vi "ClientTestVI.vi"() -> ()   [LabVIEW 2018, in "TCP_Client.lvlib"]
uses:
  TCP_Client/TCP_Client.lvclass
  TCP_Client.lvlib
panel:
  out "Waveform Graph":dbl[](graph)
  in  "stop":bool
  out "error out":errorcluster
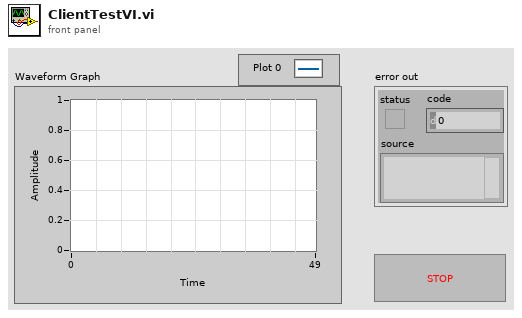
[diagram p1: front panel]
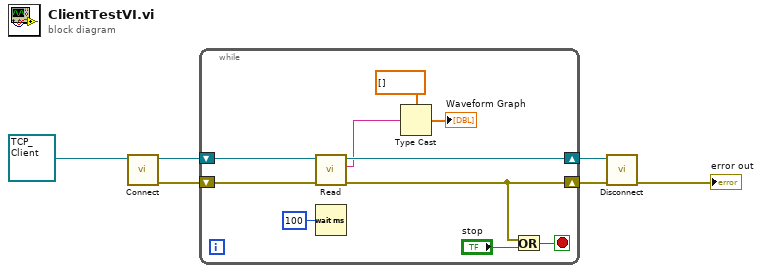
[diagram p0: block diagram]
diagram:
  n1 = call-dynamic "Connect.vi"("TCP_Client in"=refnum<class "TCP_Client.lvclass"> refnum) -> ("error out"=w4:errorcluster, "TCP_Client out"=w5:refnum<class "TCP_Client.lvclass">)  [unwired: 9 in]
  n2 = while {
    shift-right: [w14] -> w3
    shift-left: w5 -> [w16]
    shift-right: [w13] -> w2
    shift-left: w4 -> [w15]
    stop <- w11 stop-if-true
    n3 = call-dynamic "Read.vi"("error in (no error)"=w15, "TCP_Client in"=w16) -> ("error out"=w13:errorcluster, "Message"=w8:string, "TCP_Client out"=w14:refnum<class "TCP_Client.lvclass">)  [unwired: 7 in]
    n4 = Wait (ms)(milliseconds to wait=u32 100) -> ()  [unwired: 1 out]
    n5 = Type Cast(type=dbl[] [] ("chart"), x=w8) -> (*(type *) &x=→"Waveform Graph":dbl[])
    n6 = Or(x=w13, y="stop") -> (x .or. y?=w11:bool)
  }
  n7 = call-dynamic "Disconnect.vi"("error in (no error)"=w2, "TCP_Client in"=w3) -> ("error out"=→"error out":errorcluster)  [unwired: 8 in, 1 out]
